vi "initialise.vi"(8 "error in (no error)":errorcluster, 11 "CameraNetworkController in":refnum<class "CameraNetworkController.lvclass">) -> (0 "error out":errorcluster, 3 "CameraNetworkController out":refnum<class "CameraNetworkController.lvclass">)   [LabVIEW 2011, in "Hardware.lvlib" / "HWControllers.lvlib" / "CameraNetworkController.lvclass"]
uses:
  CameraNetworkController.lvclass
  CameraNetworkController.lvclass/CameraNetworkController.ctl
  NetworkClient/NetworkServer.lvclass
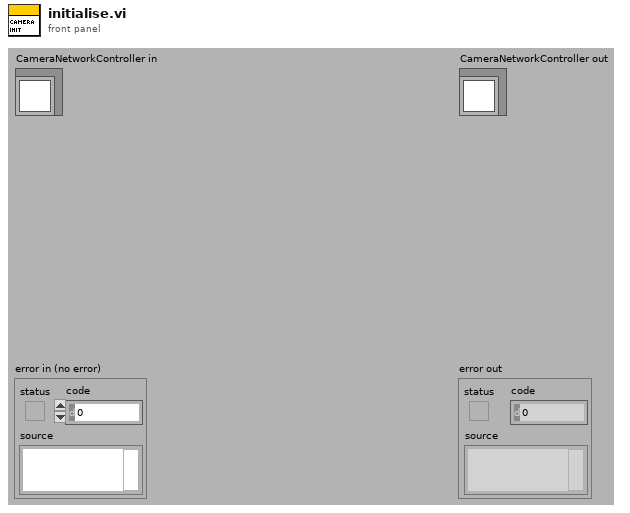
[diagram p1: front panel]
types:
  T1 = cluster{"Message":enum16{"Idle", "initialise", "configureAcquisition", "setTemperature", "getTemperature", "start", "stop", "sendImage", "close", "error", "ExitApp"}, "Data":variant}
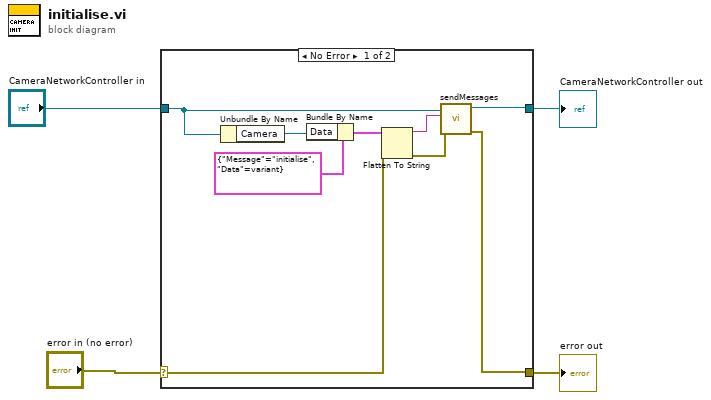
[diagram p0: block diagram]
diagram:
  n1 = case shown="No Error" "error in (no error)" {
    selector: "error in (no error)" -> [w8 w15]
    tunnel: [w5 w15] -> w3
    tunnel: [w12 w14] -> w1
    tunnel: "CameraNetworkController in" -> [w13 w14]
    frame No Error {
      n2 = Unbundle By Name(w13) -> ("Camera"=w10:refnum<class "Camera.lvclass">)
      n3 = Bundle By Name(cluster=T1 {"Message"=enum."initialise", "Data"=variant}, "Data"=w10) -> (w9:T1)
      n4 = Flatten To String(anything=w9, error in (no error)=w8) -> (data string=w6:string, error out=w7:errorcluster)  [unwired: 3 out]
      n5 = call "sendMessages.vi"("error in (no error)"=w7, "messageString"=w6, "NetworkClient in"=w13) -> ("error out"=w5:errorcluster, "NetworkClient out"=w12:refnum<class "CameraNetworkController.lvclass">)  [unwired: 7 in]
    }
    frame Error {
    }
  }
  "error out" <- w3
  "CameraNetworkController out" <- w1
